vi "Four Track - Main.vi"() -> ()   [LabVIEW 2014]
uses:
  <vilib>/myRIO/Common/Instrument Driver Framework/Utilities/typedefs/Analog Scaling Constants.ctl
  <vilib>/myRIO/Common/Instrument Driver Framework/Utilities/typedefs/Generic FPGA Reference.ctl
  <vilib>/myRIO/Common/Instrument Driver Framework/Utilities/typedefs/myRIO v1.0 Reference.ctl
  <vilib>/myRIO/Common/Instrument Driver Framework/Utilities/typedefs/Hardware Version Enum.ctl
  <vilib>/myRIO/Common/Instrument Driver Framework/Utilities/typedefs/myRIO Generic Hardware Reference.ctl
  <vilib>/userdefined/High Color/nirio_resource_hc.ctl
  <vilib>/myRIO/Instrument Drivers/Onboard IO/AudioOut Block/AudioOut Block.lvlib
  <vilib>/myRIO/Common/Instrument Driver Framework/myRIO v1.0/AudioOut Block/typedefs/AudioOut Block Channels Enum.ctl
  <vilib>/myRIO/Common/Instrument Driver Framework/myRIO v1.0/AudioOut Block/typedefs/AudioOut Block Channels List.ctl
  <vilib>/myRIO/Instrument Drivers/Onboard IO/AudioOut Block/typedefs/AudioOut Block Reference.ctl
  <vilib>/myRIO/Instrument Drivers/Onboard IO/AudioOut Block/vis/myRIO AudioOut N Samples Open.xnode
  <vilib>/myRIO/Common/Instrument Driver Framework/myRIO v1.0/AudioOut Block/vis/myRIO v1.1 Open Throughput AudioOut (N Samples).vi
  <vilib>/myRIO/Common/Instrument Driver Framework/myRIO v1.0/AudioIn Block/typedefs/AudioIn Block Channels Enum.ctl
  <vilib>/myRIO/Common/Instrument Driver Framework/myRIO v1.0/AudioIn Block/typedefs/AudioIn Block Channels List.ctl
  <vilib>/myRIO/Instrument Drivers/Onboard IO/AudioIn Block/typedefs/AudioIn Block Reference.ctl
  <vilib>/myRIO/Instrument Drivers/Onboard IO/AudioIn Block/AudioIn Block.lvlib
  <vilib>/myRIO/Instrument Drivers/Onboard IO/AudioIn Block/vis/myRIO AudioIn N Samples Open.xnode
  <vilib>/myRIO/Common/Instrument Driver Framework/myRIO v1.0/AudioIn Block/vis/myRIO v1.1 Open Throughput AudioIn (N Samples).vi
  Sub VIs/Audio/Controls/playback state.ctl
  Audio In.ctl
  4 Track Audio.ctl
  Track Effects Settings.ctl
  Track Volume Settings.ctl
  Track Settings.ctl
  Sub VIs/Audio/Controls/Delay Controls.ctl
  Track Controls.ctl
  Playback Controls.ctl
  File Controls.ctl
panel:
  out "x*y":dbl
  out "Numeric":dbl
  out "Right":dbl[](graph)
  out "Left":dbl[](graph)
  in  "stop":bool
  out "Playback State":T1
  out "error out":errorcluster
  in  "error in (no error)":errorcluster
  in  "Track Controls":T2={"Track 0"={"Effects Settings"={"Delay"=4.86522497566e-313, "Delay 2"=4.86522497566e-313}, "Volume Settings"={"Mute"=FALSE, "Solo"=FALSE, "Record"=FALSE, "Pan"=4.86522497566e-313, "Volume"=4.86522497566e-313}}, "Track 1"={"Effects Settings"={"Delay"=0.0, "Delay 2"=0.0}, "Volume Settings"={"Mute"=FALSE, "Solo"=FALSE, "Record"=FALSE, "Pan"=0.0, "Volume"=0.0}}, "Track 2"={"Effects Settings"={"Delay"=0.0, "Delay 2"=0.0}, "Volume Settings"={"Mute"=FALSE, "Solo"=FALSE, "Record"=FALSE, "Pan"=0.0, "Volume"=0.0}}, "Track 3"={"Effects Settings"={"Delay"=0.0, "Delay 2"=0.0}, "Volume Settings"={"Mute"=FALSE, "Solo"=FALSE, "Record"=FALSE, "Pan"=0.0, "Volume"=0.0}}} {"Track 3"."Volume Settings"."Volume" scale=0.001..5.0; "Track 3"."Volume Settings"."Pan" scale=0.0..1.0; "Track 3"."Effects Settings"."Delay 2" scale=0.0..10.0; "Track 3"."Effects Settings"."Delay" scale=0.0..10.0; "Track 2"."Volume Settings"."Volume" scale=0.001..5.0; "Track 2"."Volume Settings"."Pan" scale=0.0..1.0; "Track 2"."Effects Settings"."Delay 2" scale=0.0..10.0; "Track 2"."Effects Settings"."Delay" scale=0.0..10.0; "Track 1"."Volume Settings"."Volume" scale=0.001..5.0; "Track 1"."Volume Settings"."Pan" scale=0.0..1.0; "Track 1"."Effects Settings"."Delay 2" scale=0.0..10.0; "Track 1"."Effects Settings"."Delay" scale=0.0..10.0; "Track 0"."Volume Settings"."Volume" scale=0.001..5.0; "Track 0"."Volume Settings"."Pan" scale=0.0..1.0; "Track 0"."Effects Settings"."Delay 2" scale=0.0..10.0; "Track 0"."Effects Settings"."Delay" scale=0.0..10.0}
  in  "Playback Controls":T6
  in  "File Controls":T7
  in  "Master Volume Settings":T5={"Mute"=FALSE, "Solo"=FALSE, "Record"=FALSE, "Pan"=0.5, "Volume"=0.0} {"Volume" scale=0.001..5.0; "Pan" scale=0.0..1.0}
  in  "Delay Settings":T8 {"Wet/Dry" scale=0.0..1.0}
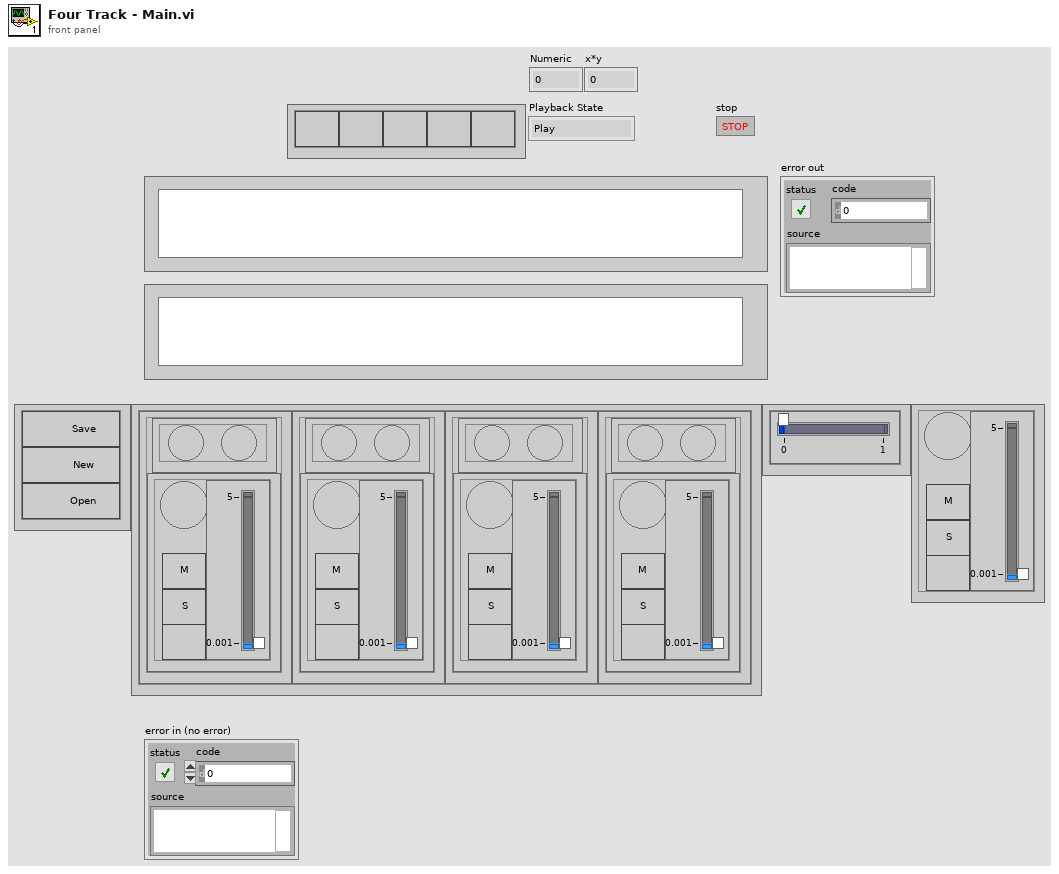
[diagram p1: front panel]
types:
  T1 = typedef "playback state.ctl" = enum16{"Play", "Record", "Stop", "Pause", "Rewind"}
  T2 = typedef "Track Controls.ctl" = cluster{"Track 0":T3, "Track 1":T3, "Track 2":T3, "Track 3":T3}
  T3 = typedef "Track Settings.ctl" = cluster{"Effects Settings":T4, "Volume Settings":T5}
  T4 = typedef "Track Effects Settings.ctl" = cluster{"Delay":dbl, "Delay 2":dbl}
  T5 = typedef "Track Volume Settings.ctl" = cluster{"Mute":bool, "Solo":bool, "Record":bool, "Pan":dbl, "Volume":dbl}
  T6 = typedef "Playback Controls.ctl" = cluster{"Play Button":bool, "Record Button":bool, "Media Stop Button":bool, "Pause Button":bool, "Skip Back Button":bool}
  T7 = typedef "File Controls.ctl" = cluster{"Save Button":bool, "New Button":bool, "Open Button":bool}
  T8 = typedef "Delay Controls.ctl" = cluster{"Wet/Dry":dbl}
  T9 = typedef "4 Track Audio.ctl" = cluster{"Track 0":T10, "Track 1":T10, "Track 2":T10, "Track 3":T10}
  T10 = typedef "Audio In.ctl" = cluster{"AudioIn/Left (N Samples)":dbl[], "AudioIn/Right (N Samples)":dbl[]}
  T11 = typedef "AudioOut Block.lvlib/AudioOut Block Reference.ctl" = cluster{"myRIO Reference":T12, "AudioOut (N Samples) Channels List":T16, "AudioOut (N Samples) Scaling Constants List":T18[]}
  T12 = typedef "myRIO Generic Hardware Reference.ctl" = cluster{"myRIO Model":T13, "myRIO Hardware Reference":T14}
  T13 = typedef "Hardware Version Enum.ctl" = enum16{"Unknown", "myRIO-1900", "myRIO-1950"}
  T14 = typedef "myRIO v1.0 Reference.ctl" = cluster{"Generic FPGA Reference":T15, "Allow multiple opens":bool}
  T15 = typedef "Generic FPGA Reference.ctl" = refnum<k20>
  T16 = typedef "AudioOut Block Channels List.ctl" = T17[]
  T17 = typedef "AudioOut Block Channels Enum.ctl" = enum16{"Not Connected", "AudioOut/Left (N Samples)", "AudioOut/Right (N Samples)"}
  T18 = typedef "Analog Scaling Constants.ctl" = cluster{"LSB Weight (Volts)":dbl, "Offset (Volts)":dbl, "Signed?":bool}
  T19 = typedef "AudioIn Block.lvlib/AudioIn Block Reference.ctl" = cluster{"myRIO Reference":T12, "AudioIn (N Samples) Channels List":T20, "AudioIn (N Samples) Scaling Constants List":T18[]}
  T20 = typedef "AudioIn Block Channels List.ctl" = T21[]
  T21 = typedef "AudioIn Block Channels Enum.ctl" = enum16{"Not Connected", "AudioIn/Left (N Samples)", "AudioIn/Right (N Samples)"}
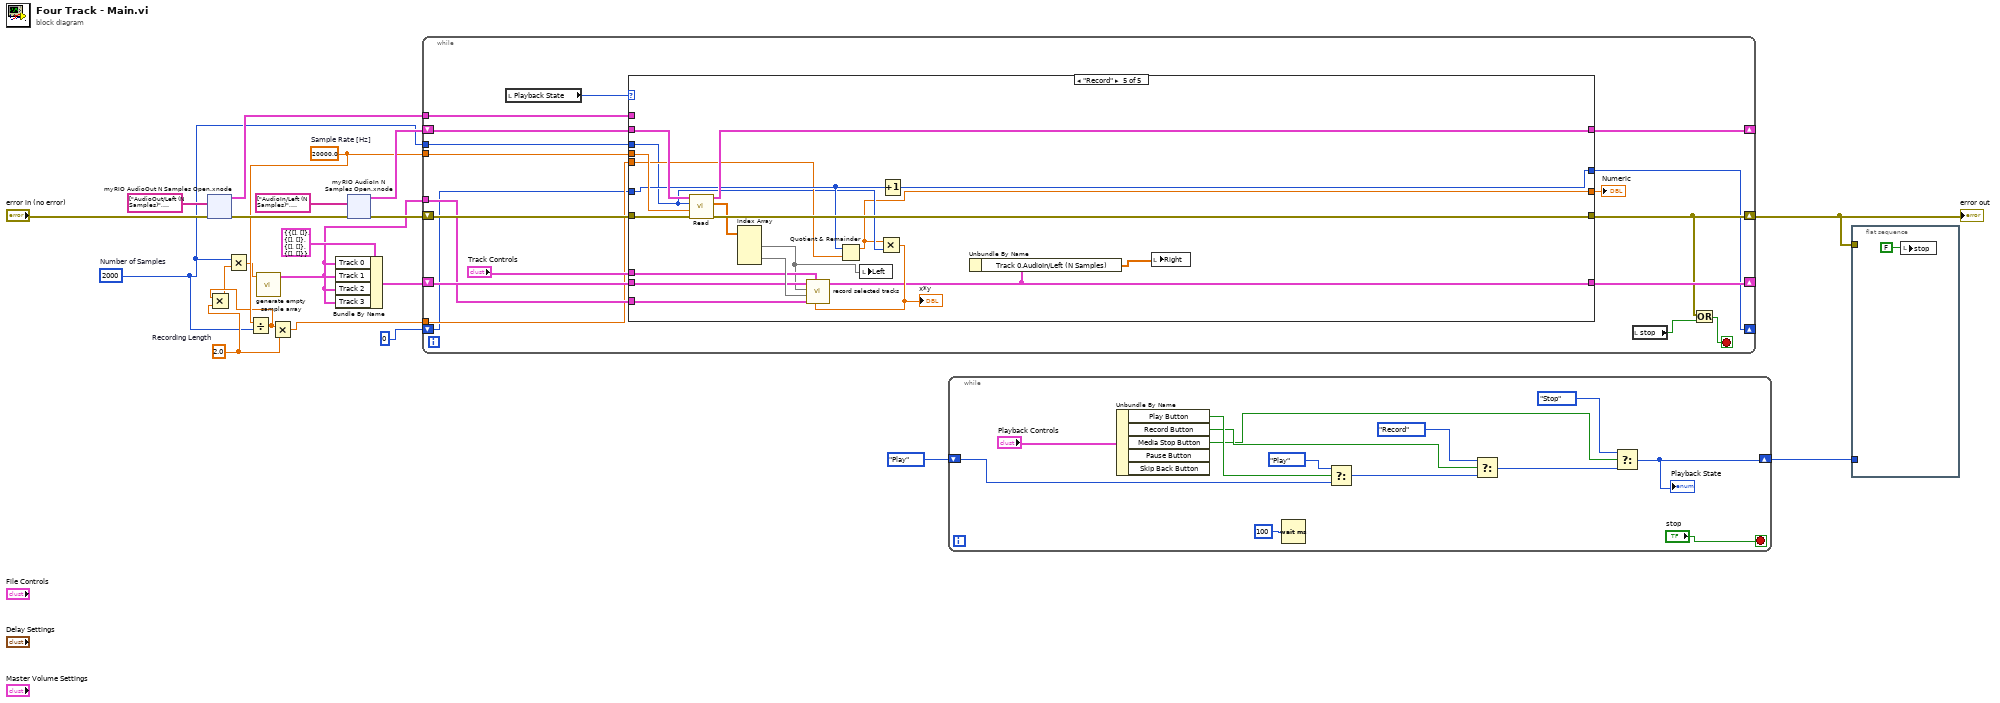
[diagram p0: block diagram]
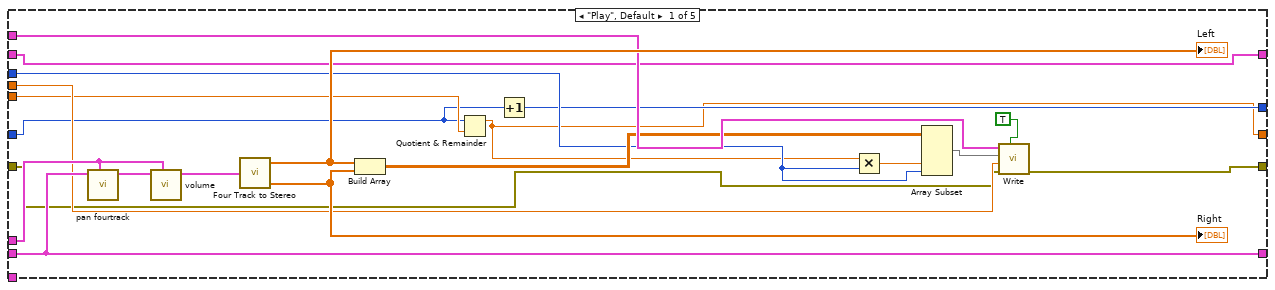
[diagram p2: hidden frame]
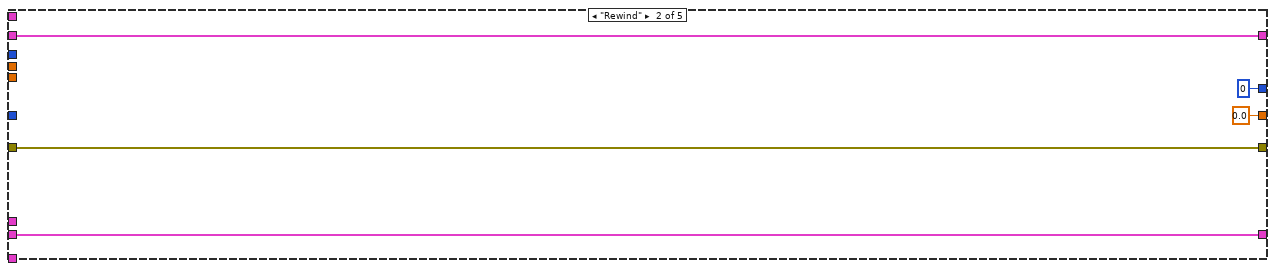
[diagram p3: hidden frame]
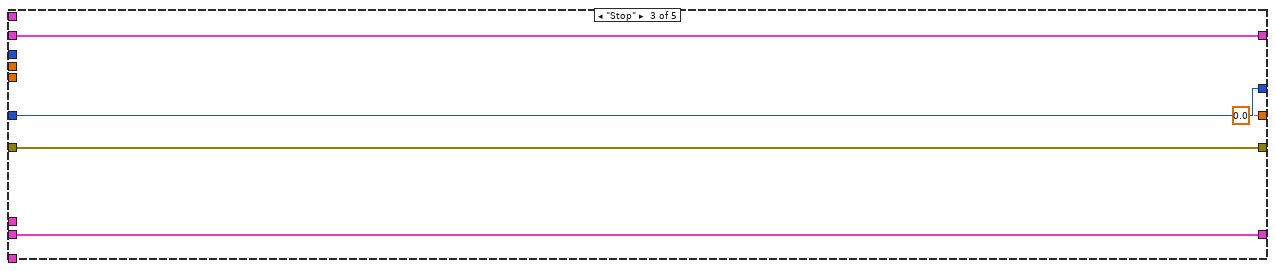
[diagram p4: hidden frame]
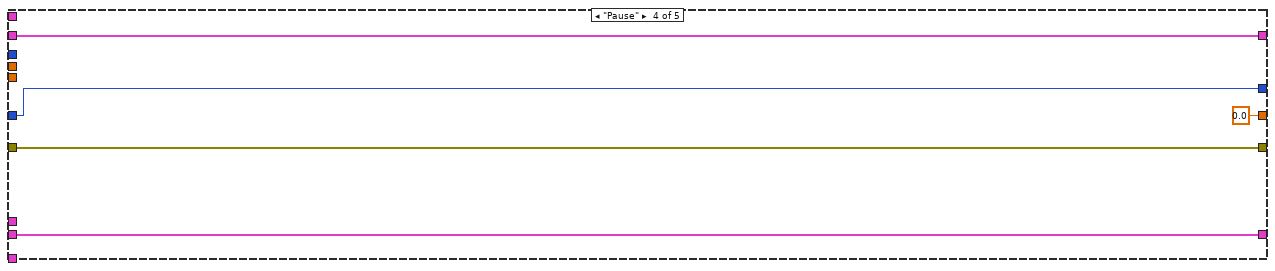
[diagram p5: hidden frame]
diagram:
  w6 = 2.0  # Recording Length
  w2 = u32 2000  # Number of Samples
  w8 = 20000.0  # Sample Rate [Hz]
  n1 = xnode "myRIO AudioOut N Samples Open.xnode"("error in (no error)"="error in (no error)", "Channel Names"=tag[] ["AudioOut/Left (N Samples)", "AudioOut/Right (N Samples)"]) -> ("error out"=w19:errorcluster, "AudioOut (N Samples) Ref Out"=w16:T11)  [unwired: 1 in]
  n2 = Divide(x=w8, y=w2) -> (x/y=w5:dbl)
  n3 = Multiply(x=w5, y=w6) -> (x*y=w4:dbl)
  n4 = Multiply(x=w2, y=w4) -> (x*y=w3:dbl)
  n5 = call "generate empty sample array.vi"("Numeric"=w3) -> ("output cluster"=w11:T10)  [unwired: 10 in]
  n6 = Multiply(x=w5, y=w6) -> (x*y=w7:dbl)
  n7 = Bundle By Name(cluster=T9 {"Track 0"={"AudioIn/Left (N Samples)"=[], "AudioIn/Right (N Samples)"=[]}, "Track 1"={"AudioIn/Left (N Samples)"=[], "AudioIn/Right (N Samples)"=[]}, "Track 2"={"AudioIn/Left (N Samples)"=[], "AudioIn/Right (N Samples)"=[]}, "Track 3"={"AudioIn/Left (N Samples)"=[], "AudioIn/Right (N Samples)"=[]}} ("4-Track Audio out"), "Track 0"=w11, "Track 1"=w11, "Track 2"=w11, "Track 3"=w11) -> (w10:T9)
  n8 = xnode "myRIO AudioIn N Samples Open.xnode"("error in (no error)"=w19, "Channel Names"=tag[] ["AudioIn/Left (N Samples)", "AudioIn/Right (N Samples)"]) -> ("error out"=w15:errorcluster, "AudioIn (N Samples) Ref Out"=w17:T19)  [unwired: 1 in]
  n9 = while {
    shift-right: [w34] -> _
    shift-left: w10 -> [w35]
    tunnel: w2 -> [w38]
    tunnel: w8 -> [w37]
    tunnel: w16 -> [w33]
    shift-right: [w26] -> w14
    shift-left: w15 -> [w32]
    tunnel: w11 -> [w30]
    shift-right: [w29] -> _
    shift-left: w17 -> [w39]
    tunnel: w7 -> [w28]
    shift-right: [w23] -> _
    shift-left: 0 -> [w24]
    stop <- w25 stop-if-true
    n10 = local read "Playback State"() -> (w31:T1)
    n11 = case shown="\"Record\"" w31 {
      tunnel: w39 -> [w47 w62 w67 w72 w93]
      tunnel: w38 -> [w48 _ _ _ w80]
      tunnel: w37 -> [w53 _ _ _ w92]
      tunnel: "Track Controls" -> [w58 _ _ _ w90]
      tunnel: w35 -> [w54 w64 w69 w74 w89]
      tunnel: [w54 w64 w69 w74 w76] -> w34
      tunnel: w33 -> [w50 _ _ _ _]
      tunnel: w32 -> [w52 w63 w68 w73 w88]
      tunnel: [w51 w63 w68 w73 w87] -> w26
      tunnel: w30 -> [_ _ _ _ w85]
      tunnel: [w47 w62 w67 w72 w84] -> w29
      tunnel: w28 -> [w46 _ _ _ w81]
      tunnel: w24 -> [w42 _ w66 w71 w82]
      tunnel: [w41 0 w66 w71 w83] -> w23
      tunnel: [w40 0.0 0.0 0.0 w78] -> w22
      frame "Play", Default {
        n12 = call "pan fourtrack.vi"("Track Controls"=w58, "4-Track Audio in"=w54) -> ("4-Track Audio out"=w59:T9)  [unwired: 9 in]
        n13 = call "volume.vi"("Track Controls"=w58, "4-Track Audio in"=w59) -> ("4-Track Audio out"=w57:T9)  [unwired: 9 in]
        n14 = call "Four Track to Stereo.vi"("4-Track Audio In"=w57) -> ("Right Out"=w55:dbl[], "Left Out"=w56:dbl[])  [unwired: 3 in]
        "Left" <- w56
        "Right" <- w55
        n15 = Build Array(w56, w55) -> (w49:dbl[][])
        n16 = Quotient & Remainder(x=w42, y=w46) -> (x-y*floor(x/y)=w40:dbl)  [unwired: 1 out]
        n17 = Increment(x=w42) -> (x+1=w41:i32)
        n18 = Multiply(x=w40, y=w48) -> (x*y=w45:dbl)
        n19 = Array Subset(array=w49, index (col)=w45, length (col)=w48) -> (w43:dbl[][])  [unwired: 2 in]
        n20 = call <vilib>:"Write.vi"("Wait Until Done?"=TRUE, "error in (no error)"=w52, "Sample Rate [Hz]"=w53, "Values"=w43, "AudioOut (N Samples) Ref In"=w50) -> ("error out"=w51:errorcluster)  [unwired: 5 in, 1 out]
      }
      frame "Rewind" {
      }
      frame "Stop" {
      }
      frame "Pause" {
      }
      frame "Record" {
        n21 = call <vilib>:"Read.vi"("error in (no error)"=w88, "Sample Rate [Hz]"=w92, "Number of Samples"=w80, "AudioIn (N Samples) Ref In"=w93) -> ("error out"=w87:errorcluster, "Values"=w86:dbl[][], "AudioIn (N Samples) Ref Out"=w84:T19)  [unwired: 5 in]
        n22 = Index Array(array=w86) -> (element #1=w77:dbl[], element #2=w91:dbl[])  [unwired: 4 in]
        n23 = Quotient & Remainder(x=w82, y=w81) -> (x-y*floor(x/y)=w78:dbl)  [unwired: 1 out]
        n24 = local write "Left"(w77) -> ()
        n25 = Multiply(x=w78, y=w80) -> (x*y=w79:dbl)
        "x*y" <- w79
        n26 = call "record selected tracks.vi"("index"=w79, "Track Controls"=w90, "Blank Track"=w85, "AudioIn/Right (N Samples)"=w91, "AudioIn/Left (N Samples)"=w77, "4-Track Audio in"=w89) -> ("4-Track Audio out"=w76:T9)  [unwired: 5 in]
        n27 = Increment(x=w82) -> (x+1=w83:i32)
        n28 = Unbundle By Name(w76) -> ("Track 0.AudioIn/Left (N Samples)"=w75:dbl[])
        n29 = local write "Right"(w75) -> ()
      }
    }
    "Numeric" <- w22
    n30 = local read "stop"() -> (w27:bool)
    n31 = Or(x=w26, y=w27) -> (x .or. y?=w25:bool)
  }
  "error out" <- w14
  n32 = while {
    shift-right: [w95] -> w9
    shift-left: playback_state."Play" ("Playback State") -> [w102]
    stop <- "stop" stop-if-true
    n33 = Unbundle By Name("Playback Controls") -> ("Play Button"=w104:bool, "Record Button"=w100:bool, "Media Stop Button"=w97:bool)  [unwired: 2 out]
    n34 = Wait (ms)(milliseconds to wait=u32 100) -> ()  [unwired: 1 out]
    n35 = Select(t=playback_state."Play" ("Playback State"), s=w104, f=w102) -> (s? t:f=w101:T1)
    n36 = Select(t=playback_state."Record", s=w100, f=w101) -> (s? t:f=w98:T1)
    n37 = Select(t=playback_state."Stop", s=w97, f=w98) -> (s? t:f=w95:T1)
    "Playback State" <- w95
  }
  n38 = flat-sequence {
    tunnel: w14 -> [_]
    tunnel: w9 -> [_]
    frame #0 {
      n39 = local write "stop"(FALSE ("stop")) -> ()
    }
  }
